vi "CheckWatchdogTimer.vi"(3 "ROS":T1, 4 "itteration":i32, 5 "LogPath in":path) -> ()   [LabVIEW 2014]
doc: "Checks the watchdog timer to close unused nodes"
uses:
  <userlib>/ROS for LabVIEW Software.lnk/ROS/Code/SubVIs/_ROSControl.ctl
  <userlib>/ROS for LabVIEW Software.lnk/ROS/Code/SubVIs/_ROSDirection.ctl
  <userlib>/ROS for LabVIEW Software.lnk/ROS/Code/_ROSDefinition.vi
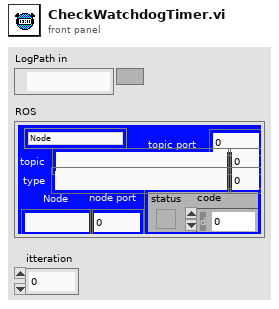
[diagram p1: front panel]
types:
  T1 = typedef "_ROSControl.ctl" = cluster{"topic port":u16, "Node":string, "topic":string, "type":string, "node port":u16, "error ":errorcluster, "Direction":T2, "Update (ms)":u16, "FIFO size":u16}
  T2 = typedef "_ROSDirection.ctl" = enum16{"Node", "Publisher", "Subscriber", "ServiceClient", "ServiceProvider"}
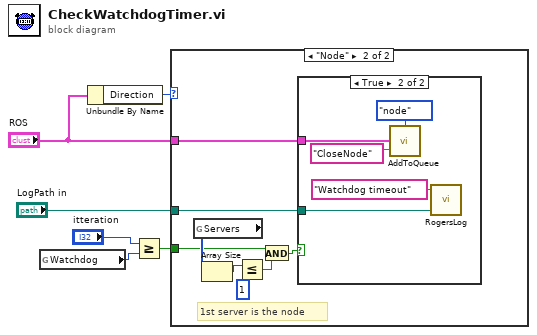
[diagram p0: block diagram]
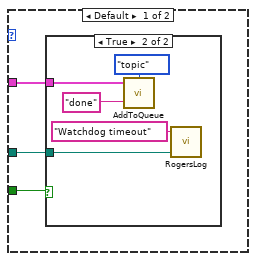
[diagram p2: hidden frame]
diagram:
  n1 = global read "_ROSDefinition.vi" "Watchdog"() -> (w3:i32)
  n2 = Unbundle By Name("ROS") -> ("Direction"=w2:T2)
  n3 = Greater Or Equal?(x="itteration", y=w3) -> (x >= y?=w5:bool)
  n4 = case shown="\"Node\"" w2 {
    tunnel: "ROS" -> [w9 w22]
    tunnel: "LogPath in" -> [w8 w21]
    tunnel: w5 -> [w7 w19]
    frame Default {
      n5 = case shown="True" w7 {
        tunnel: w8 -> [_ w13]
        tunnel: w9 -> [_ w12]
        frame False {
        }
        frame True {
          n6 = call <userlib>:"AddToQueue.vi"("Cmd"="done" ("element"), "ROS"=w12, "Type"=enum16{"topic", "node", "ToFIFO", "ToWrite"}."topic") -> ()  [unwired: 2 in, 1 out]
          n7 = call <userlib>:"RogersLog.vi"("Text to add"="Watchdog timeout", "LogPath in"=w13) -> ()  [unwired: 3 in, 2 out]
        }
      }
    }
    frame "Node" {
      # "1st server is the node"
      n8 = global read "_ROSDefinition.vi" "Servers"() -> (w20:u16[])
      n9 = Array Size(array=w20) -> (size(s)=w16:i32)
      n10 = Less Or Equal?(x=w16, y=1) -> (x <= y?=w18:bool)
      n11 = And(x=w19, y=w18) -> (x .and. y?=w17:bool)
      n12 = case shown="True" w17 {
        tunnel: w21 -> [_ w26]
        tunnel: w22 -> [_ w25]
        frame False {
        }
        frame True {
          n13 = call <userlib>:"AddToQueue.vi"("Cmd"="CloseNode" ("element"), "ROS"=w25, "Type"=enum16{"topic", "node", "ToFIFO", "ToWrite"}."node") -> ()  [unwired: 2 in, 1 out]
          n14 = call <userlib>:"RogersLog.vi"("Text to add"="Watchdog timeout", "LogPath in"=w26) -> ()  [unwired: 3 in, 2 out]
        }
      }
    }
  }
